vi "Insulation_ST5520.vi"(7 "lbl log std":string, 8 "errin":errorcluster, 11 "Refnum VISA en entrée":refnum<visa-resource-name>) -> (0 "error out":errorcluster caption="sortie d'erreur", 1 "PASS?":bool, 2 "R iso(MOhm)":dbl, 3 "MSG":string, 4 "LOG Html":string[](array[string]), 5 "Status":T2(ring), 6 "LOG STD":string, 9 "sous-chaîne précédente":string, 10 "Rin":string)   [LabVIEW 2020]
uses:
  D:/CODE/Equipment/09 ST5520/Public/Lower/Config Measure/ST5520 Set Measurement Configuration.vi
  D:/CODE/Equipment/09 ST5520/Public/Lower/Comparator/ST5520 Set Comparator.vi
  D:/CODE/Equipment/09 ST5520/Public/Lower/Testing Status/ST5520 Start.vi
  D:/CODE/Equipment/09 ST5520/Public/Lower/Testing Status/ST5520 State.vi
  D:/CODE/Equipment/09 ST5520/Public/Lower/Measurement/ST5520 Read Resistance.vi
  D:/CODE/Equipment/09 ST5520/Public/Lower/Testing Status/ST5520 Stop.vi
  <userlib>/Hioki ST5520/ST5520.lvlib
panel:
  out "Judgement Result":T1(ring)
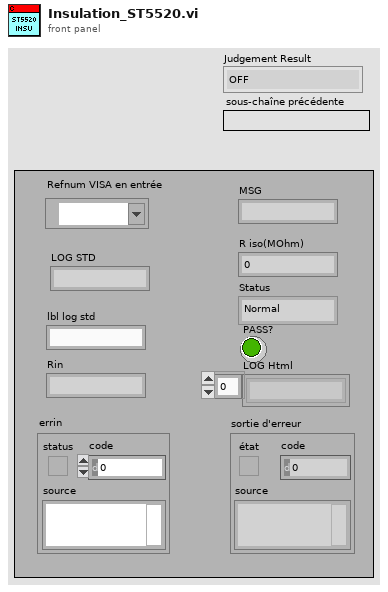
[diagram p1: front panel]
types:
  T1 = enum16{"OFF", "NOCOMP", "DELAY", "PASS", "UFAIL", "LFAIL", "ULFAIL"}
  T2 = enum16{"Normal", "Over Flow", "Under Flow", "Error"}
  T3 = cluster{"Baud Rate":u32, "Frequency":enum8{"AUTO", "50", "60"}, "Resistance Range":cluster{"Range":enum16{"2M", "20M", "200M", "2000M", "4000M", "AUTO"}, "Set Check Range Change if AUTO":enum16{"ON", "OFF"}}, "Voltage":u16, "Timing":cluster{"Measurement Speed":enum16{"FAST", "SLOW"}, "Timer":cluster{"Set/Unset":enum8{"Set", "Unset"}, "Duration":dbl}, "Delay":cluster{"Set/Unset":enum8{"Set", "Unset"}, "Duration":dbl}}, "Beep":enum8{"PASS", "FAIL", "OFF", "END"}, "Mode":enum8{"CONTINUE", "PASSSTOP", "FAILSTOP", "SEQUENCE"}, "Upper Limit":cluster{"ON/OFF":enum8{"ON", "OFF"}, "Limit Value":dbl}, "Lower Limit":cluster{"ON/OFF":enum8{"ON", "OFF"}, "Limit Value":dbl}}
  T4 = cluster{"Range":enum16{"2M", "20M", "200M", "2000M", "4000M", "AUTO"}, "Set Check Range Change if AUTO":enum16{"ON", "OFF"}}
  T5 = cluster{"Measurement Speed":enum16{"FAST", "SLOW"}, "Timer":cluster{"Set/Unset":enum8{"Set", "Unset"}, "Duration":dbl}, "Delay":cluster{"Set/Unset":enum8{"Set", "Unset"}, "Duration":dbl}}
  T6 = enum8{"CONTINUE", "PASSSTOP", "FAILSTOP", "SEQUENCE"}
  T7 = cluster{"ON/OFF":enum8{"ON", "OFF"}, "Limit Value":dbl}
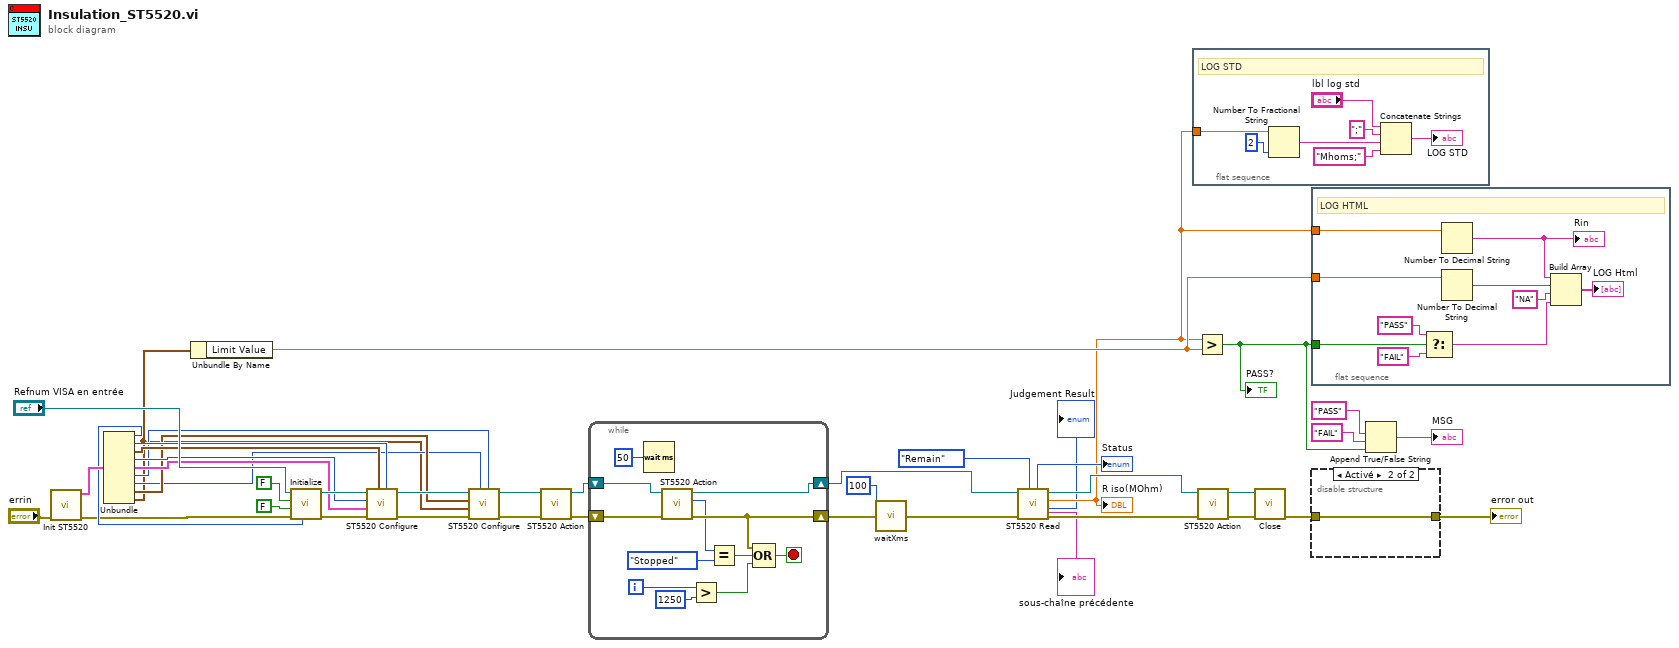
[diagram p0: block diagram]
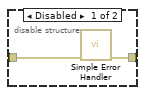
[diagram p2: hidden frame]
diagram:
  n1 = call <userlib>:"Init ST5520.vi"("error in (no error)"="errin") -> ("error out"=w22:errorcluster, "Cluster Paramètres fichier Ini"=w25:T3)  [unwired: 9 in]
  n2 = Unbundle(w25) -> ("Baud Rate"=w24:u32, "Frequency"=w20:enum8{"AUTO", "50", "60"}, "Resistance Range"=w19:T4, "Voltage"=w21:u16, "Timing"=w18:T5, "Beep"=w15:enum8{"PASS", "FAIL", "OFF", "END"}, "Mode"=w16:T6, "Upper Limit"=w17:T7, "Lower Limit"=w14:T7)
  n3 = Unbundle By Name(w14) -> ("Limit Value"=w9:dbl)
  n4 = call "Initialize.vi"("VISA resource name"="Refnum VISA en entrée", "ID Query (True)"=FALSE, "Reset (True)"=FALSE, "error in (no error)"=w22, "Baud Rate"=w24) -> ("VISA resource name out"=w29:refnum<visa-resource-name>, "error out"=w28:errorcluster)  [unwired: 4 in]
  n5 = call-poly "ST5520 Configure.vi"("Frequency"=w20, "Resistance Range"=w19, "error in (no error)"=w28, "Timing"=w18, "Voltage"=w21, "VISA resource name"=w29) -> ("error out"=w32:errorcluster, "VISA resource name out"=w30:refnum<visa-resource-name>)  [unwired: 4 in]
  n6 = call-poly "ST5520 Configure.vi"("Beep"=w15, "Mode"=w16, "error in (no error)"=w32, "Lower Limit"=w14, "Upper Limit"=w17, "VISA resource name"=w30) -> ("error out"=w33:errorcluster, "VISA resource name out"=w31:refnum<visa-resource-name>)  [unwired: 4 in]
  n7 = call-poly "ST5520 Action.vi"("error in (no error)"=w33, "VISA resource name"=w31) -> ("error out"=w37:errorcluster, "VISA resource name out"=w38:refnum<visa-resource-name>)  [unwired: 8 in]
  n8 = while {
    shift-right: [w55] -> w43
    shift-left: w38 -> [w52]
    shift-right: [w49] -> w7
    shift-left: w37 -> [w51]
    i -> [w45]
    stop <- w48 stop-if-true
    n9 = Wait (ms)(milliseconds to wait=u32 50) -> ()  [unwired: 1 out]
    n10 = call-poly "ST5520 Action.vi"("error in (no error)"=w51, "VISA resource name"=w52) -> ("error out"=w49:errorcluster, "State"=w44:enum8{"Stopped", "Testing ", "Discharging"}, "VISA resource name out"=w55:refnum<visa-resource-name>)  [unwired: 7 in]
    n11 = Greater?(x=w45, y=1250) -> (0:w46:bool)
    n12 = Equal?(x=w44, y=enum8{"Stopped", "Testing ", "Discharging"}."Stopped" ("State")) -> (x = y?=w50:bool)
    n13 = Compound Arithmetic op=OR(w49, w50, w46) -> (w48:bool)
  }
  n14 = call <userlib>:"waitXms.vi"("attente (ms)"=u32 100, "errin"=w7) -> ("errout"=w6:errorcluster)  [unwired: 13 in]
  n15 = call-poly "ST5520 Read.vi"("Clear Measurement"=enum16{"Remain", "Clear"}."Remain", "err in"=w6, "visa in"=w43) -> ("error out"=w39:errorcluster, "Judgement Result"=→"Judgement Result":T1, "Measured Value (MOhm)"=w8:dbl, "VISA resource name out"=w40:refnum<visa-resource-name>, "sous-chaîne précédente"=→"sous-chaîne précédente":string, "Status"=→"Status":T2)  [unwired: 3 in]
  "R iso(MOhm)" <- w8
  n16 = flat-sequence {
    tunnel: w8 -> [w59]
    frame #0 {
      # "LOG STD"
      n17 = Number To Fractional String(number=w59, precision (6)=i16 2 ("précision (6)")) -> (F-format string=w62:string)  [unwired: 2 in]
      n18 = Concatenate Strings("lbl log std", ";" ("chaîne"), w62, "Mhoms;" ("chaîne")) -> (→"LOG STD":string)
    }
  }
  n19 = Greater?(x=w8, y=w9) -> (0:w11:bool)
  "PASS?" <- w11
  n20 = call-poly "ST5520 Action.vi"("error in (no error)"=w39, "VISA resource name"=w40) -> ("error out"=w35:errorcluster, "VISA resource name out"=w36:refnum<visa-resource-name>)  [unwired: 8 in]
  n21 = call "Close.vi"("error in (no error)"=w35, "VISA resource name"=w36) -> ("error out"=w34:errorcluster)  [unwired: 9 in]
  n22 = flat-sequence {
    tunnel: w11 -> [w65]
    tunnel: w9 -> [w64]
    tunnel: w8 -> [w63]
    frame #0 {
      # "LOG HTML"
      n23 = Select(t="PASS", s=w65, f="FAIL") -> (s? t:f=w66:string)
      n24 = Number To Decimal String(number=w63) -> (decimal integer string=w72:string)  [unwired: 1 in]
      "Rin" <- w72
      n25 = Number To Decimal String(number=w64) -> (decimal integer string=w71:string)  [unwired: 1 in]
      n26 = Build Array(w72, w71, "NA" ("élément"), w66) -> (→"LOG Html":string[])
    }
  }
  n27 = disable-structure shown="Activé" {
    disable-tunnel: w34 -> [w74 w75]
    disable-tunnel: [w73 w75] -> w26
    frame Disabled {
      n28 = call <vilib>:"Simple Error Handler.vi"("error in (no error)"=w74) -> ("error out"=w73:errorcluster)  [unwired: 4 in, 4 out]
    }
    frame Enabled {
    }
  }
  "error out" <- w26
  n29 = Append True/False String(1:w11, 2:"FAIL" ("chaîne faux"), 3:"PASS" ("chaîne vrai")) -> (0:→"MSG":string)  [unwired: 1 in]
